vi "Get Variable Reference by Name from Local Machine.vi"(7 "Access Type":T1, 8 "error in":errorcluster, 10 "Search":string) -> (0 "error out":errorcluster, 2 "Found":bool, 3 "Variable References Out":refnum<k21>[](array[refnum]))   [LabVIEW 2017, in "Shared Variables Library.lvlib"]
doc: "Get reference to a local shared variable, by searching for the shared variable using it's name.\n\nReturns an array of references, as multiple variables may contain similar string in their names."
uses:
  Shared Variables Library.lvlib
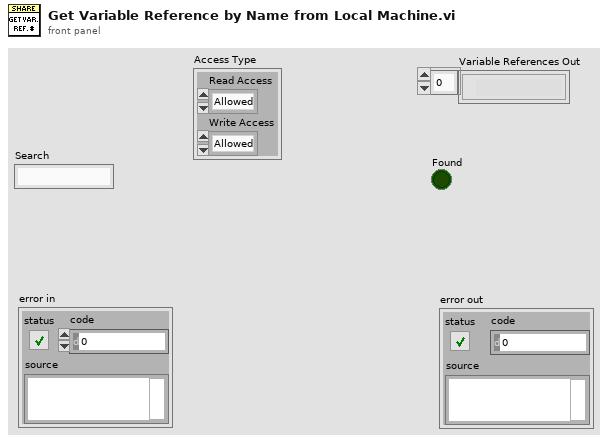
[diagram p1: front panel]
types:
  T1 = cluster{"Read Access":enum8{"Allowed", "Required", "Denied"}, "Write Access":enum8{"Allowed", "Required", "Denied"}}
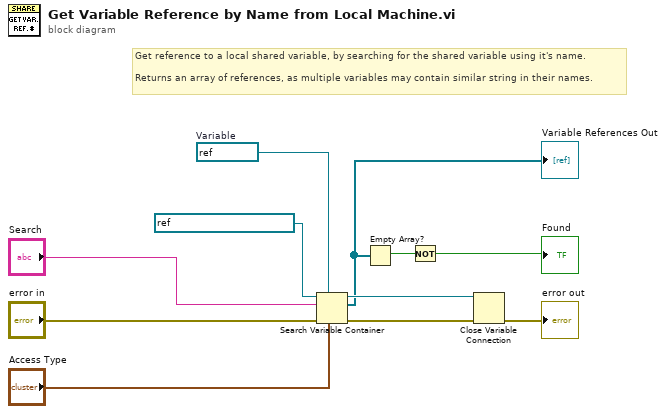
[diagram p0: block diagram]
diagram:
  w2 = refnum<k21> refnum  # Variable
  # "Get reference to a local shared variable, by searching for the shared variable using it's name.\n\nReturns an array of references, as multiple variables may contain similar string in their names."
  n1 = Search Variable Container(6:"Access Type", 7:w2, 8:"error in", 10:"Search", 11:refnum<k21> "ni.var.psp://localhost" ("container refnum in")) -> (0:w7:errorcluster, 2:w6:refnum<k21>[], 3:w8:refnum<k21>)  [unwired: 1 in]
  "Variable References Out" <- w6
  n2 = Empty Array?(array=w6) -> (empty?=w5:bool)
  n3 = Not(x=w5) -> (.not. x?=→"Found":bool)
  n4 = Close Variable Connection(8:w7, 11:w8) -> (0:→"error out":errorcluster)
